vi "COM.vi"(2 "y in":dbl, 3 "x in":dbl, 4 "Kantenlänge":dbl, 5 "Array":dbl[][](array[numeric])) -> (0 "Y out":dbl, 1 "X out":dbl)   [LabVIEW 2017]
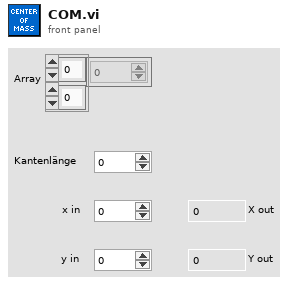
[diagram p1: front panel]
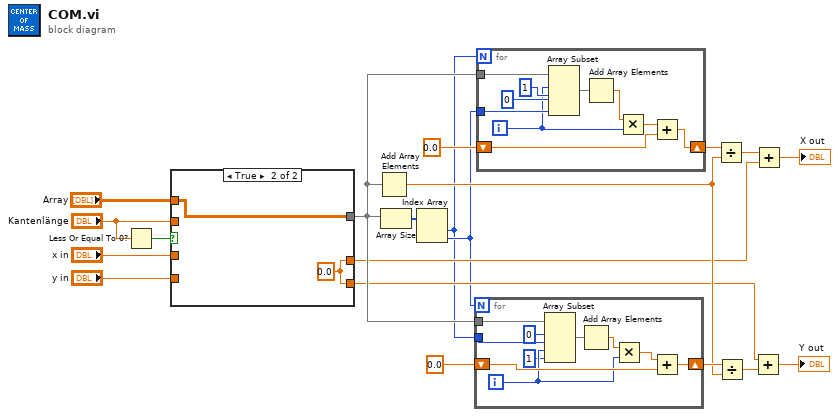
[diagram p0: block diagram]
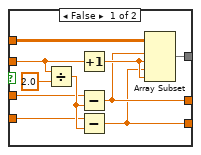
[diagram p2: hidden frame]
diagram:
  n1 = Less Or Equal To 0?(x="Kantenlänge") -> (x <= 0?=w8:bool)
  n2 = case shown="True" w8 {
    tunnel: "x in" -> [w27 _]
    tunnel: "y in" -> [w26 _]
    tunnel: "Array" -> [w25 w32]
    tunnel: [w24 w32] -> w9
    tunnel: "Kantenlänge" -> [w23 _]
    tunnel: [w22 w31] -> w6
    tunnel: [w21 w31] -> w5
    frame False {
      n3 = Divide(x=w23, y=2.0) -> (x/y=w28:dbl)
      n4 = Increment(x=w23) -> (x+1=w29:dbl)
      n5 = Subtract(x=w27, y=w28) -> (x-y=w22:dbl)
      n6 = Subtract(x=w26, y=w28) -> (x-y=w21:dbl)
      n7 = Array Subset(array=w25, index (row)=w22, length (row)=w29, index (col)=w21, length (col)=w29) -> (w24:dbl[][])
    }
    frame True {
      w31 = 0.0
    }
  }
  n8 = Add Array Elements(numeric array=w9) -> (sum=w16:dbl)
  n9 = Array Size(array=w9) -> (size(s)=w20:i32[])
  n10 = Index Array(array=w20) -> (element #1=w1:i32, element #2=w2:i32)  [unwired: 2 in]
  n11 = for {
    N: w2 -> [_]
    tunnel: w9 -> [w42]
    shift-right: [w37] -> w17
    shift-left: 0.0 -> [w38]
    tunnel: w1 -> [w35]
    i -> [w34]
    n12 = Array Subset(array=w42, index (row)=0 ("index"), length (row)=w35, index (col)=w34, length (col)=1 ("length")) -> (w41:dbl[][])
    n13 = Add Array Elements(numeric array=w41) -> (sum=w40:dbl)
    n14 = Multiply(x=w40, y=w34) -> (x*y=w39:dbl)
    n15 = Add(x=w39, y=w38) -> (x+y=w37:dbl)
  }
  n16 = for {
    N: w1 -> [_]
    tunnel: w9 -> [w52]
    shift-right: [w47] -> w18
    shift-left: 0.0 -> [w48]
    tunnel: w2 -> [w44]
    i -> [w43]
    n17 = Array Subset(array=w52, index (row)=w43, length (row)=1 ("length"), index (col)=0 ("index"), length (col)=w44) -> (w51:dbl[][])
    n18 = Add Array Elements(numeric array=w51) -> (sum=w50:dbl)
    n19 = Multiply(x=w50, y=w43) -> (x*y=w49:dbl)
    n20 = Add(x=w49, y=w48) -> (x+y=w47:dbl)
  }
  n21 = Divide(x=w18, y=w16) -> (x/y=w14:dbl)
  n22 = Divide(x=w17, y=w16) -> (x/y=w15:dbl)
  n23 = Add(x=w5, y=w15) -> (x+y=→"Y out":dbl)
  n24 = Add(x=w14, y=w6) -> (x+y=→"X out":dbl)
